vi "NiFpga_HdlFifo32_WriteI8.vi"(6 "timeout":u32, 7 "error in (no error)":errorcluster, 8 "data in":i8[](array[numeric]), 9 "fifo number":u32, 10 "fpga vi reference in":refnum<k20>) -> (0 "error out":errorcluster, 1 "empty elements remaining":u64, 3 "fpga vi reference out":refnum<k20>)   [LabVIEW 2023]
doc: "Dynamically reads the register at the provided offset. Set check for errors to true to check for errors such as if the register offset is invalid or if the register is running in an external clock domain that might not be running."
uses:
  NiFpga.dll
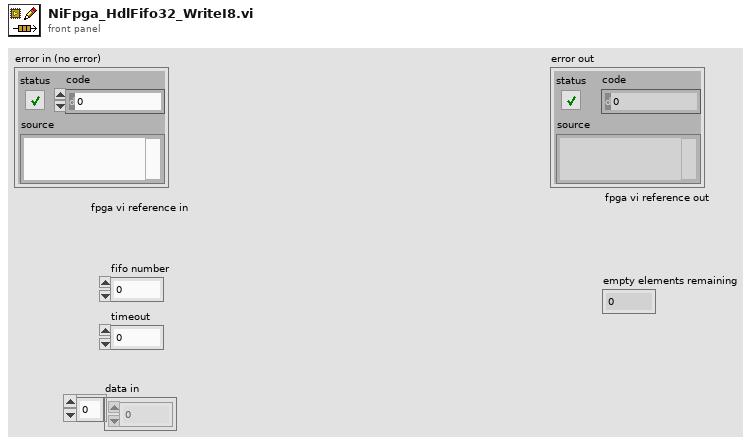
[diagram p1: front panel]
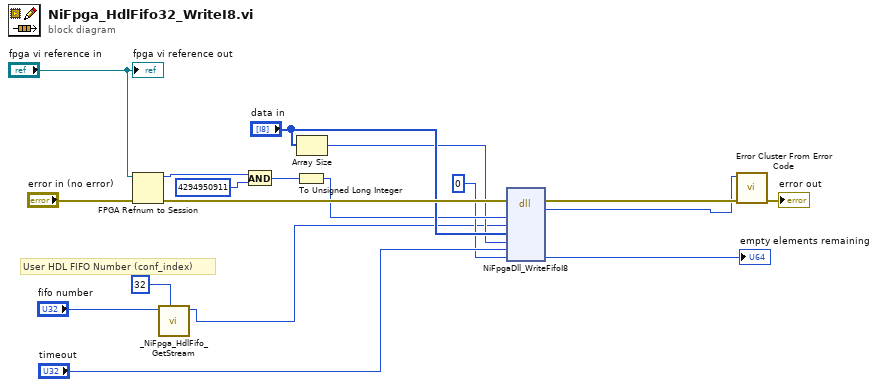
[diagram p0: block diagram]
diagram:
  # "User HDL FIFO Number (conf_index)"
  n1 = FPGA Refnum to Session(4:"error in (no error)", 7:"fpga vi reference in") -> (0:w13:errorcluster, 3:w15:u64)
  n2 = call "_NiFpga_HdlFifo_GetStream.vi"("NUM_DMA_CHANNELS"=u32 32, "Fifo Number"="fifo number") -> ("Fifo Stream"=w2:u32)  [unwired: 9 in]
  n3 = And(x=w15, y=u64 4294950911) -> (x .and. y?=w7:u64)
  n4 = To Unsigned Long Integer(number=w7) -> (unsigned 32bit integer=w6:u32)
  n5 = Array Size(array="data in") -> (size(s)=w5:i32)
  n6 = dll-call lib="NiFpga.*" fn="NiFpgaDll_WriteFifoI8"(error in=w13, "session"=w6, "fifo"=w2, "data"="data in", "numberOfElements"=w5, "timeout"="timeout", "emptyElementsRemainining"=u64 0) -> (error out=w12:errorcluster, "return type"=w11:i32, "emptyElementsRemainining"=→"empty elements remaining":u64)  [unwired: 7 in, 1 out]
  n7 = call <vilib>:"Error Cluster From Error Code.vi"("error in (no error)"=w12, "error code (0)"=w11) -> ("error out"=→"error out":errorcluster)  [unwired: 7 in]
  "fpga vi reference out" <- "fpga vi reference in"
